vi "VG-select_graph_dataformat.vi"(9 "Graph Data":T1, 11 "data format":T2) -> (1 "Graph Data out":T1)   [LabVIEW 2020, in "VG-VNA_GUI.lvlib" / "VG-VNA_GUI.lvclass"]
uses:
  VG-VNA_GUI.lvclass
  VG-data_format_selector.ctl
  VG-graph_data.ctl
panel:
  out "Numeric":i32
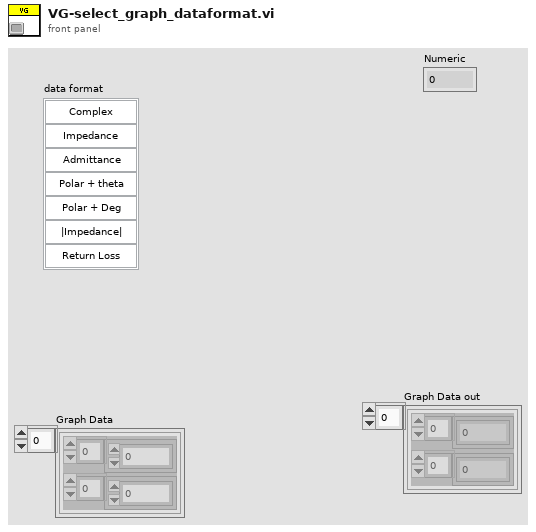
[diagram p1: front panel]
types:
  T1 = typedef "VG-VNA_GUI.lvlib/VG-VNA_GUI.lvclass/VG-graph_data.ctl" = cluster{u64[], dbl[]}[]
  T2 = typedef "VG-VNA_GUI.lvlib/VG-VNA_GUI.lvclass/VG-data_format_selector.ctl" = cluster{"Complex":bool, "Impedance":bool, "Admittance":bool, "Polar":bool, "Polar Deg":bool, "|Impedance|":bool, "Return Loss":bool}
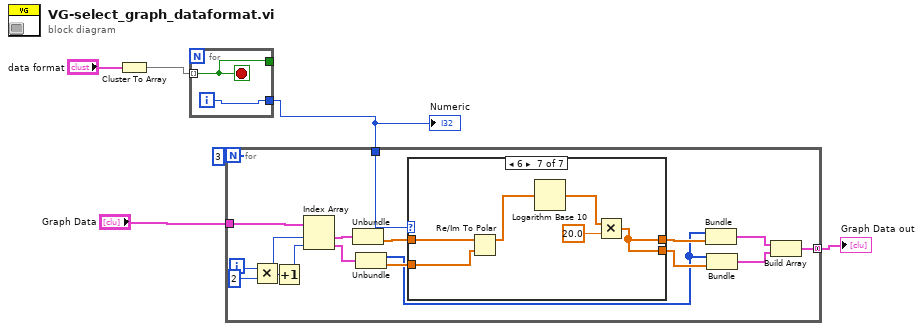
[diagram p0: block diagram]
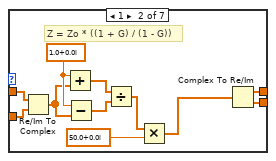
[diagram p3: hidden frame]
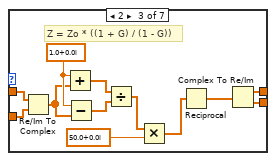
[diagram p4: hidden frame]
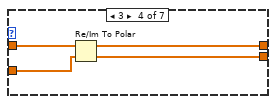
[diagram p5: hidden frame]
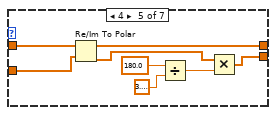
[diagram p6: hidden frame]
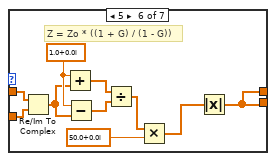
[diagram p7: hidden frame]
diagram:
  n1 = Cluster To Array(cluster="data format") -> (array=w5:bool[])
  n2 = for {
    tunnel: w5 -> [w7] mode=indexing
    tunnel: [w8] -> w1
    tunnel: [w7] -> _
    i -> [w8]
    stop <- w7 stop-if-true
  }
  "Numeric" <- w1
  n3 = for {
    N: 3 -> [_]
    tunnel: w1 -> [w24]
    tunnel: "Graph Data" -> [w21]
    tunnel: [w9] -> w2 mode=concatenating
    i -> [w20]
    n4 = Multiply(x=w20, y=2) -> (x*y=w17:i32)
    n5 = Increment(x=w17) -> (x+1=w18:i32)
    n6 = Index Array(array=w21, index #1=w17, index #2=w18) -> (element #1=w16:cluster{u64[], dbl[]}, element #2=w15:cluster{u64[], dbl[]})
    n7 = Unbundle(w16) -> (w23:dbl[])  [unwired: 1 out]
    n8 = Unbundle(w15) -> (w12:u64[], w14:dbl[])
    n9 = case shown="6" w24 {
      tunnel: w23 -> [w26 w29 w42 w52 w60 w66 w76]
      tunnel: [w26 w31 w44 w51 w59 w62 w72] -> w22
      tunnel: w14 -> [w25 w28 w41 w53 w61 w65 w77]
      tunnel: [w25 w30 w43 w50 w54 w62 w72] -> w13
      frame 0, Default {
      }
      frame 1 {
        w37 = cdb 1.0+0.0i ("x")
        # "Z = Zo * ((1 + G) / (1 - G))"
        n10 = Re/Im To Complex(1:w28, 2:w29) -> (0:w27:cdb[])
        n11 = Add(x=w37, y=w27) -> (x+y=w36:cdb[])
        n12 = Subtract(x=w37, y=w27) -> (x-y=w35:cdb[])
        n13 = Divide(x=w36, y=w35) -> (x/y=w34:cdb[])
        n14 = Multiply(x=w34, y=cdb 50.0+0.0i) -> (x*y=w32:cdb[])
        n15 = Complex To Re/Im(x + iy=w32) -> (x=w31:dbl[], y=w30:dbl[])
      }
      frame 2 {
        w49 = cdb 1.0+0.0i ("x")
        # "Z = Zo * ((1 + G) / (1 - G))"
        n16 = Re/Im To Complex(1:w41, 2:w42) -> (0:w40:cdb[])
        n17 = Add(x=w49, y=w40) -> (x+y=w48:cdb[])
        n18 = Subtract(x=w49, y=w40) -> (x-y=w47:cdb[])
        n19 = Divide(x=w48, y=w47) -> (x/y=w46:cdb[])
        n20 = Multiply(x=w46, y=cdb 50.0+0.0i) -> (x*y=w39:cdb[])
        n21 = Reciprocal(x=w39) -> (1/x=w38:cdb[])
        n22 = Complex To Re/Im(x + iy=w38) -> (x=w44:dbl[], y=w43:dbl[])
      }
      frame 3 {
        n23 = Re/Im To Polar(2:w53, 3:w52) -> (0:w50:dbl[], 1:w51:dbl[])
      }
      frame 4 {
        n24 = Re/Im To Polar(2:w61, 3:w60) -> (0:w55:dbl[], 1:w59:dbl[])
        n25 = Divide(x=180.0, y=3.141592653589793) -> (x/y=w56:dbl)
        n26 = Multiply(x=w55, y=w56) -> (x*y=w54:dbl[])
      }
      frame 5 {
        w71 = cdb 1.0+0.0i ("x")
        # "Z = Zo * ((1 + G) / (1 - G))"
        n27 = Re/Im To Complex(1:w65, 2:w66) -> (0:w64:cdb[])
        n28 = Add(x=w71, y=w64) -> (x+y=w70:cdb[])
        n29 = Subtract(x=w71, y=w64) -> (x-y=w69:cdb[])
        n30 = Divide(x=w70, y=w69) -> (x/y=w68:cdb[])
        n31 = Multiply(x=w68, y=cdb 50.0+0.0i) -> (x*y=w63:cdb[])
        n32 = Absolute Value(x=w63) -> (abs(x)=w62:dbl[])
      }
      frame 6 {
        n33 = Re/Im To Polar(2:w77, 3:w76) -> (1:w73:dbl[])  [unwired: 1 out]
        n34 = Logarithm Base 10(1:w73) -> (0:w75:dbl[])
        n35 = Multiply(x=w75, y=20.0) -> (x*y=w72:dbl[])
      }
    }
    n36 = Bundle(w12, w22) -> (w11:cluster{u64[], dbl[]})  [unwired: 1 in]
    n37 = Bundle(w12, w13) -> (w10:cluster{u64[], dbl[]})  [unwired: 1 in]
    n38 = Build Array(w11, w10) -> (w9:cluster{u64[], dbl[]}[])
  }
  "Graph Data out" <- w2
